vi "BioMapT2mWriter(Mapping).vi"(8 "error in":errorcluster, 9 "SpecLength":u16, 10 "mzArray":dbl[](array[numeric])=[0.0, 1.0, 0.0], 11 "image file path":path) -> (0 "error out":errorcluster)   [LabVIEW 2012]
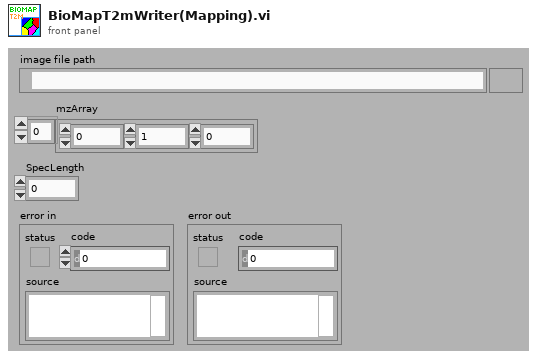
[diagram p1: front panel]
types:
  T1 = enum16{"big-endian, network order", "native, host order", "little-endian"}
  T2 = enum16{"open", "replace", "create", "open or create", "replace or create", "replace or create with confirmation"}
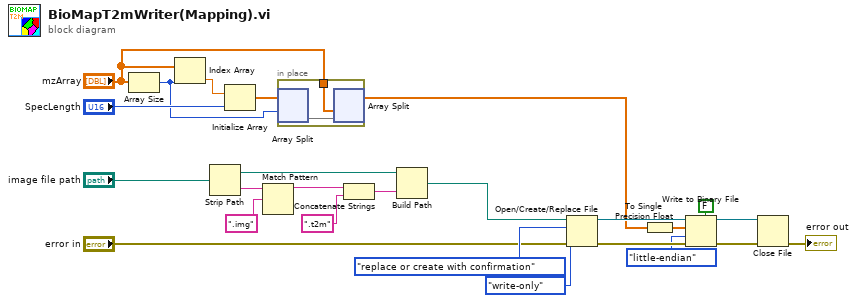
[diagram p0: block diagram]
diagram:
  n1 = Array Size(array="mzArray") -> (size(s)=w3:i32)
  n2 = Index Array(array="mzArray", index=w3) -> (element=w5:dbl)
  n3 = Strip Path(path="image file path") -> (stripped path=w11:path, name=w15:string)
  n4 = Initialize Array(w5, "SpecLength") -> (w4:dbl[])
  n5 = Match Pattern(string=w15, regular expression=".img" ("string")) -> (before substring=w14:string)  [unwired: 1 in, 3 out]
  n6 = in-place {
    in-place-border: "mzArray" -> [w27]
    n7 = in-place-split #1(w4, w3) -> (w26:dbl[])  [unwired: 1 out]
    n8 = in-place-split #1(w27, w26) -> (w1:dbl[])  [unwired: 1 out]
  }
  n9 = Concatenate Strings(w14, ".t2m" ("string")) -> (w12:string)
  n10 = Build Path(base path=w11, name or relative path=w12) -> (appended path=w10:path)
  n11 = Open/Create/Replace File(file path (use dialog)=w10, error in="error in", operation (0:open)=T2."replace or create with confirmation", access (0:read/write)=enum16{"read/write", "read-only", "write-only"}."write-only") -> (refnum out=w23:refnum<file>, error out=w20:errorcluster)  [unwired: 2 in, 1 out]
  n12 = To Single Precision Float(number=w1) -> (single precision float=w25:sgl[])
  n13 = Write to Binary File(file (use dialog)=w23, data=w25, error in=w20, 5:FALSE ("prepend array or string size? (T)"), 9:T1."little-endian" ("byte order (0:big-endian, network order)")) -> (refnum out=w18:refnum<file>, error out=w19:errorcluster)  [unwired: 1 in, 1 out]
  n14 = Close File(refnum=w18, error in=w19) -> (error out=→"error out":errorcluster)  [unwired: 1 out]
